vi "Get Ctrl Refnum.vi"(8 "error in (no error)":errorcluster, 11 "Button in":refnum<class "Button.lvclass">) -> (0 "error out":errorcluster, 2 "Ctl Refnum":refnum<vi>, 3 "Button out":refnum<class "Button.lvclass">)   [LabVIEW 2020, in "Button.lvlib" / "Button.lvclass"]
uses:
  Button.lvclass
  Button.lvclass/Button.ctl
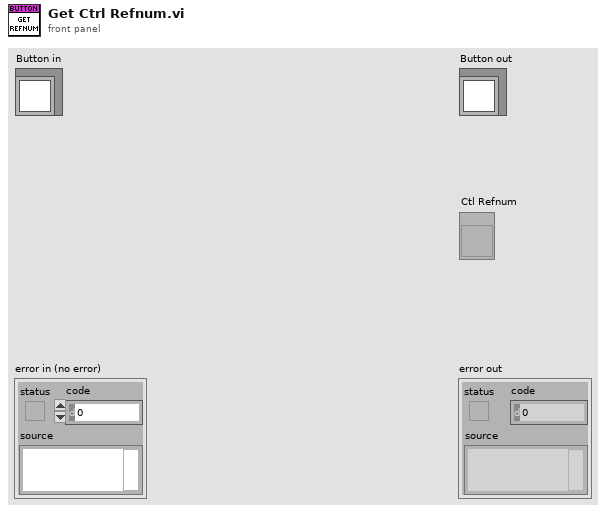
[diagram p1: front panel]
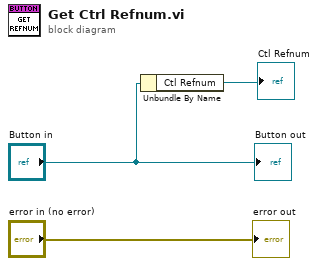
[diagram p0: block diagram]
diagram:
  n1 = Unbundle By Name("Button in") -> ("Ctl Refnum"=→"Ctl Refnum":refnum<vi>)
  "error out" <- "error in (no error)"
  "Button out" <- "Button in"
